vi "Read Measurement.vi"(8 "error in (no error)":errorcluster, 11 "VISA resource name":refnum<visa-resource-name>) -> (0 "error out":errorcluster, 2 "Data":dbl[](array[numeric]), 3 "VISA resource name out":refnum<visa-resource-name>)   [LabVIEW 2017, in "Sefram DAS220.lvlib"]
doc: "Read data from the recorder as single precision. Channel values from the array are represented as :\n<B>0 (A1) - 199 (J20)</B> : analog channels\n<B>200 (K1) - 203 (K4)</B> : digital functions channels\n<B>204 (FA1) - 243 (FJ4)</B> : functions between channels\n<B>244 (DI1) - 255 (DI12)</B> : digital channels"
uses:
  <instrlib>/Sefram DAS220/Sefram DAS220.lvlib
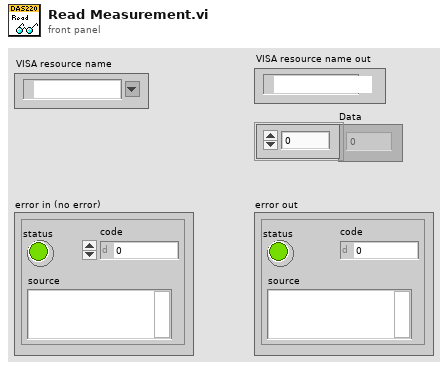
[diagram p1: front panel]
types:
  T1 = enum16{"big-endian, network order", "native, host order", "little-endian"}
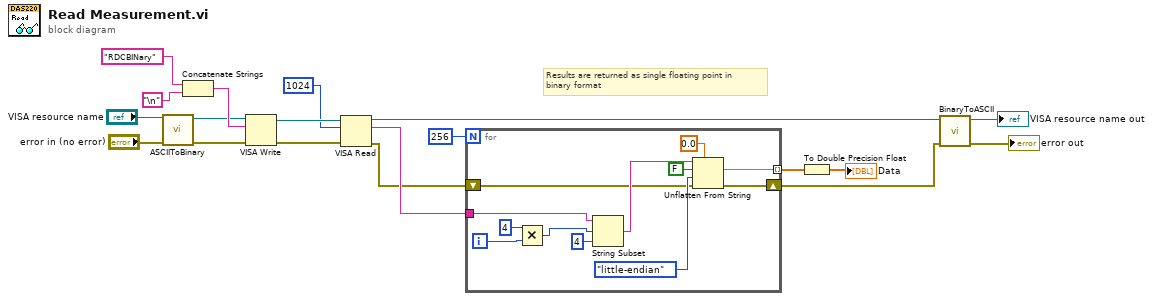
[diagram p0: block diagram]
diagram:
  # "Results are returned as single floating point in\nbinary format"
  n1 = call <instrlib>:"ASCIIToBinary.vi"("error in (no error)"="error in (no error)", "VISA resource name"="VISA resource name") -> ("error out"=w5:errorcluster, "VISA resource name"=w7:refnum<visa-resource-name>)  [unwired: 8 in]
  n2 = Concatenate Strings("RDCBINary" ("write buffer"), "\n") -> (w18:string)
  n3 = VISA Write(VISA resource name=w7, write buffer=w18, error in (no error)=w5) -> (VISA resource name out=w16:refnum<visa-resource-name>, error out=w15:errorcluster)  [unwired: 1 out]
  n4 = VISA Read(VISA resource name=w16, byte count=u32 1024, error in (no error)=w15) -> (VISA resource name out=w4:refnum<visa-resource-name>, read buffer=w14:string, error out=w12:errorcluster)  [unwired: 1 out]
  n5 = for {
    N: 256 -> [_]
    tunnel: [w25] -> w11 mode=indexing
    tunnel: w14 -> [w23]
    shift-right: [w21] -> w2
    shift-left: w12 -> [w22]
    i -> [w31]
    n6 = Multiply(x=4, y=w31) -> (x*y=w24:i32)
    n7 = String Subset(string=w23, offset (0)=w24, length (rest)=4 ("length (rest)")) -> (substring=w29:string)
    n8 = Unflatten From String(type=sgl 0.0, binary string=w29, data includes array or string size? (T)=FALSE, byte order (0:big-endian, network order)=T1."little-endian", error in (no error)=w22) -> (value=w25:sgl, error out=w21:errorcluster)  [unwired: 1 out]
  }
  n9 = To Double Precision Float(number=w11) -> (double precision float=→"Data":dbl[])
  n10 = call <instrlib>:"BinaryToASCII.vi"("error in (no error)"=w2, "VISA resource name"=w4) -> ("error out"=→"error out":errorcluster, "VISA resource name"=→"VISA resource name out":refnum<visa-resource-name>)  [unwired: 8 in]
